vi "Compile Event Capture 1.0 Data.vi"(8 "error in (no error)":errorcluster, 11 "Device Item Ref in":T3 format="%.0x") -> (0 "error out":errorcluster, 2 "Event Timing Captures":T1[](array[typedef]), 3 "Device Item Ref out":T3 format="%.0x")   [LabVIEW 2013, in "Engine Simulation Toolkit System Explorer.lvlib"]
uses:
  Engine Simulation Toolkit System Explorer.lvlib
  <vilib>/NI Veristand/Custom Device API/Custom Device Item Ref.ctl
  Shared/1.0 Event Timing Capture Engine Data.ctl
  Shared/1.0 Event Timing Capture FIFO Idxs.ctl
  Shared/Constants and GUIDs.vi
  <vilib>/NI Veristand/Custom Device Tools/Custom Device Utility Library/NI VeriStand - Search for All Items by GUID.vi
  Shared/Properties.vi
  <vilib>/NI Veristand/Custom Device API/Get Item Property (String).vi
  Shared/Engine Simulation Toolkit Shared.lvlib
  <vilib>/NI Veristand/Custom Device Tools/Custom Device Utility Library/Custom Device Utility Library.lvlib
  <vilib>/NI Veristand/Custom Device API/Custom Device API.lvlib
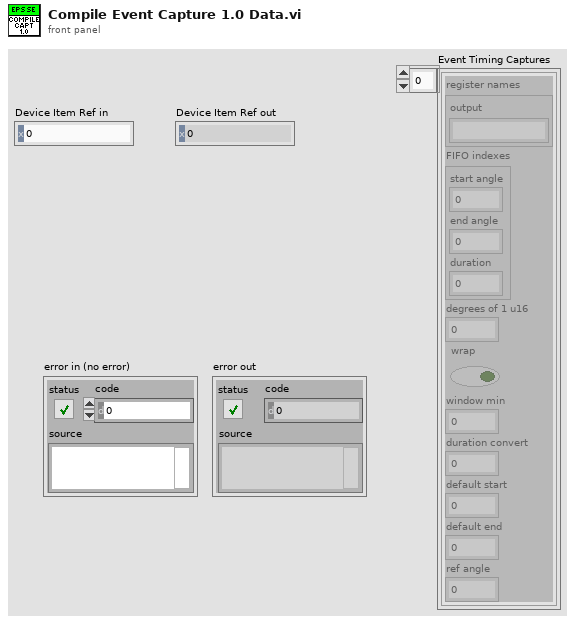
[diagram p1: front panel]
types:
  T1 = typedef "Engine Simulation Toolkit Shared.lvlib/1.0 Event Timing Capture Engine Data.ctl" = cluster{"register names":cluster{"output":string}, "FIFO indexes":T2, "degrees of 1 u16":dbl, "wrap":bool, "window min":u16, "duration convert":dbl, "default start":dbl, "default end":dbl, "ref angle":dbl}
  T2 = typedef "Engine Simulation Toolkit Shared.lvlib/1.0 Event Timing Capture FIFO Idxs.ctl" = cluster{"start angle":i32, "end angle":i32, "duration":i32}
  T3 = typedef "Custom Device API.lvlib/Custom Device Item Ref.ctl" = u64
  T4 = typedef "Engine Simulation Toolkit Shared.lvlib/Channel.ctl" = cluster{"Name":string, "Units":string, "Default":dbl, "Description":string}
  T5 = typedef "Engine Simulation Toolkit System Explorer.lvlib/Event Timing Window.ctl" = cluster{"Name":string, "Min":dbl, "Max":dbl, "Ref":dbl}
  T6 = typedef "Engine Simulation Toolkit System Explorer.lvlib/Event Timing Capture.ctl" = cluster{"Name":string, "Bitfile name":string, "Reference angle":dbl, "Default start":dbl, "Default end":dbl, "Ref Select":T7}
  T7 = typedef "Engine Simulation Toolkit System Explorer.lvlib/Event Reference Angle Selection.ctl" = enum16{"From window", "Custom"}
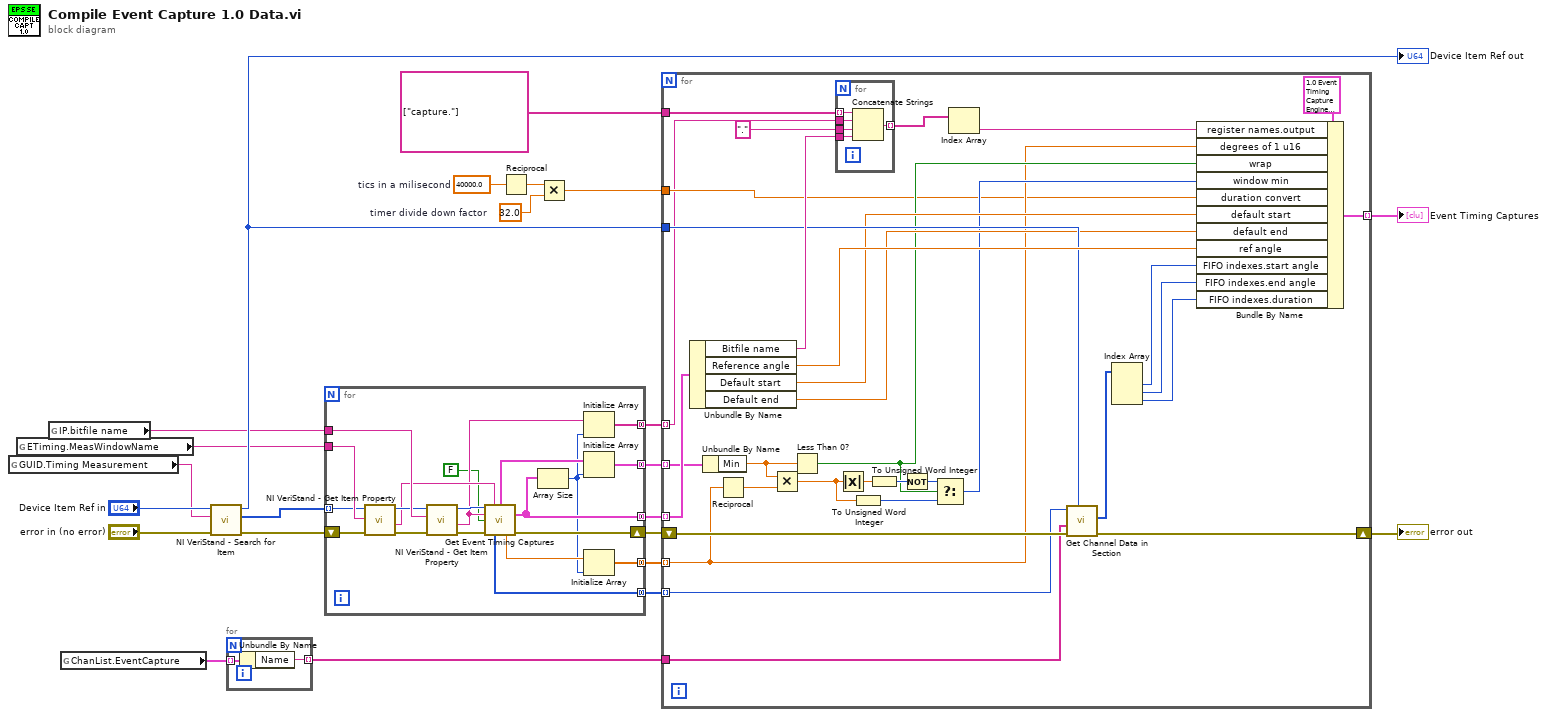
[diagram p0: block diagram]
diagram:
  w3 = 32.0  # timer divide down factor
  w5 = 40000.0  # tics in a milisecond
  n1 = global read "Constants and GUIDs.vi" "GUID.Timing Measurement"() -> (w14:string)
  n2 = global read "Properties.vi" "ETiming.MeasWindowName"() -> (w11:string)
  n3 = global read "Properties.vi" "IP.bitfile name"() -> (w10:string)
  n4 = global read "Constants and GUIDs.vi" "ChanList.EventCapture"() -> (w16:T4[])
  n5 = call-poly <vilib>:"NI VeriStand - Search for Item.vi"("error in"="error in (no error)", "Item GUID"=w14, "Section Ref in"="Device Item Ref in") -> ("error out"=w21:errorcluster, "Item Refs"=w12:T3[], "Section Ref out"=w17:T3)  [unwired: 5 in, 1 out]
  "Device Item Ref out" <- w17
  n6 = for {
    tunnel: w16 -> [w25] mode=indexing
    tunnel: [w24] -> w15 mode=indexing
    n7 = Unbundle By Name(w25) -> ("Name"=w24:string)
  }
  n8 = for {
    tunnel: w12 -> [w29] mode=indexing
    shift-right: [w40] -> w13
    shift-left: w21 -> [w45]
    tunnel: w11 -> [w42]
    tunnel: w10 -> [w41]
    tunnel: [w34] -> w9 mode=concatenating
    tunnel: [w37] -> w8 mode=concatenating
    tunnel: [w36] -> w7 mode=concatenating
    tunnel: [w33] -> w6 mode=concatenating
    tunnel: [w31] -> w1 mode=concatenating
    n9 = call-poly <vilib>:"NI VeriStand - Get Item Property.vi"("error in (no error)"=w45, "Property Name"=w42, "Item Ref in"=w29) -> ("error out"=w44:errorcluster, "Value"=w28:string, "Item Ref out"=w30:T3)  [unwired: 5 in, 1 out]
    n10 = call-poly <vilib>:"NI VeriStand - Get Item Property.vi"("error in (no error)"=w44, "Property Name"=w41, "Item Ref in"=w30) -> ("error out"=w43:errorcluster, "Value"=w27:string, "Item Ref out"=w39:T3)  [unwired: 5 in, 1 out]
    n11 = call "Get Event Timing Captures.vi"("Item Ref in"=w39, "Window"=w28, "Timing measurement"=w27, "return all captures (T)"=FALSE, "error in (no error)"=w43) -> ("window"=w35:T5, "captures"=w34:T6[], "Capture item refs"=w36:T3[], "degrees of one u16"=w38:dbl, "error out"=w40:errorcluster)  [unwired: 2 in, 4 out]
    n12 = Array Size(array=w34) -> (size(s)=w32:i32)
    n13 = Initialize Array(w27, w32) -> (w31:string[])
    n14 = Initialize Array(w35, w32) -> (w33:T5[])
    n15 = Initialize Array(w38, w32) -> (w37:dbl[])
  }
  n16 = Reciprocal(x=w5) -> (1/x=w4:dbl)
  n17 = Multiply(x=w4, y=w3) -> (x*y=w2:dbl)
  n18 = for {
    shift-right: [w66] -> w19
    shift-left: w13 -> [w70]
    tunnel: string[] ["capture."] -> [w78]
    tunnel: w15 -> [w67]
    tunnel: [w76] -> w18 mode=indexing
    tunnel: w17 -> [w68]
    tunnel: w9 -> [w75] mode=indexing
    tunnel: w8 -> [w50] mode=indexing
    tunnel: w7 -> [w69] mode=indexing
    tunnel: w6 -> [w59] mode=indexing
    tunnel: w2 -> [w48]
    tunnel: w1 -> [w46] mode=indexing
    n19 = Unbundle By Name(w75) -> ("Bitfile name"=w74:string, "Reference angle"=w71:dbl, "Default start"=w61:dbl, "Default end"=w60:dbl)
    n20 = Unbundle By Name(w59) -> ("Min"=w52:dbl)
    n21 = Reciprocal(x=w50) -> (1/x=w49:dbl)
    n22 = Multiply(x=w52, y=w49) -> (x*y=w51:dbl)
    n23 = Less Than 0?(x=w52) -> (x < 0?=w54:bool)
    n24 = for {
      tunnel: w78 -> [w83] mode=indexing
      tunnel: [w79] -> w73 mode=indexing
      tunnel: w74 -> [w82]
      tunnel: w46 -> [w81]
      tunnel: "." -> [w80]
      n25 = Concatenate Strings(w83, w81, w80, w82) -> (w79:string)
    }
    n26 = Absolute Value(x=w51) -> (abs(x)=w56:dbl)
    n27 = To Unsigned Word Integer(number=w51) -> (unsigned 16bit integer=w58:u16)
    n28 = To Unsigned Word Integer(number=w56) -> (unsigned 16bit integer=w55:u16)
    n29 = Not(x=w55) -> (.not. x?=w57:u16)
    n30 = Select(t=w57, s=w54, f=w58) -> (s? t:f=w53:u16)
    n31 = Index Array(array=w73) -> (element=w72:string)  [unwired: 1 in]
    n32 = call "Get Channel Data in Section.vi"("Custom device ref"=w68, "error in (no error)"=w70, "Channels"=w67, "Item Ref in"=w69) -> ("error out"=w66:errorcluster, "FIFO indexes"=w65:i32[])  [unwired: 3 in, 3 out]
    n33 = Index Array(array=w65) -> (element #1=w64:i32, element #2=w63:i32, element #3=w62:i32)  [unwired: 3 in]
    n34 = Bundle By Name(cluster=T1 {"register names"={"output"=""}, "FIFO indexes"={"start angle"=0, "end angle"=0, "duration"=0}, "degrees of 1 u16"=0.0, "wrap"=FALSE, "window min"=0, "duration convert"=0.0, "default start"=0.0, "default end"=0.0, "ref angle"=0.0} ("1.0.0 Event Timing Capture"), "register names.output"=w72, "degrees of 1 u16"=w50, "wrap"=w54, "window min"=w53, "duration convert"=w48, "default start"=w61, "default end"=w60, "ref angle"=w71, "FIFO indexes.start angle"=w64, "FIFO indexes.end angle"=w63, "FIFO indexes.duration"=w62) -> (w76:T1)
  }
  "error out" <- w19
  "Event Timing Captures" <- w18
